vi "getSourcedCurrent.vi"(7 "chn":string, 8 "error in (no error)":errorcluster, 11 "PowerSupply in":refnum<class "PowerSupply.lvclass">) -> (0 "error out":errorcluster, 2 "Current Limit":dbl, 3 "PowerSupply out":refnum<class "PowerSupply.lvclass">)   [LabVIEW 2023, in "swePsu.lvlib" / "PowerSupply.lvclass"]
doc: "Request the actual sourced current by the supply."
uses:
  PowerSupply.lvclass
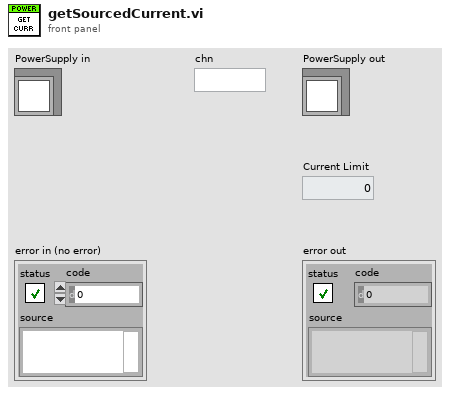
[diagram p1: front panel]
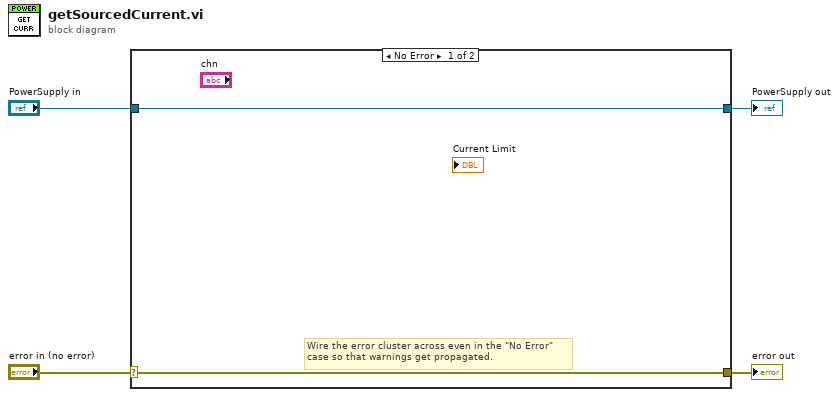
[diagram p0: block diagram]
diagram:
  n1 = case shown="No Error" "error in (no error)" {
    selector: "error in (no error)" -> [w5 w8]
    tunnel: [w5 w8] -> w3
    tunnel: [w6 w7] -> w1
    tunnel: "PowerSupply in" -> [w6 w7]
    frame No Error {
      # "Wire the error cluster across even in the \"No Error\"\ncase so that warnings get propagated."
    }
    frame Error {
    }
  }
  "error out" <- w3
  "PowerSupply out" <- w1
